vi "Memory.Error Handler.Replace String in Source.vi"(9 "offset (0)":i32, 10 "string":string, 11 "error in":errorcluster) -> (1 "new offset":i32, 3 "error out":errorcluster)   [LabVIEW 2016, in "LabVIEW Memory Manager.lvlib"]
uses:
  LabVIEW Memory Manager.lvlib
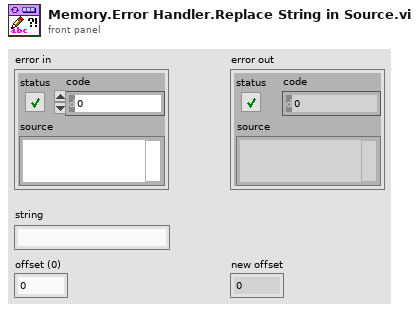
[diagram p1: front panel]
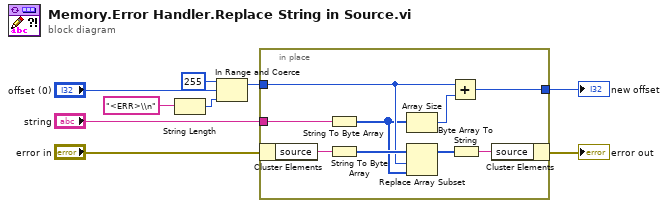
[diagram p0: block diagram]
diagram:
  n1 = String Length(string="<ERR>\\n") -> (length=w4:i32)
  n2 = In Range and Coerce(upper limit=255, x="offset (0)", lower limit=w4) -> (coerced(x)=w1:i32)  [unwired: 1 out]
  n3 = in-place {
    in-place-border: "string" -> [w15]
    in-place-border: w1 -> [w13]
    in-place-border: [w10] -> w6
    n4 = in-place-cluster #1("error in") -> ("source"=w17:string)
    n5 = String To Byte Array(string=w15) -> (unsigned byte array=w12:u8[])
    n6 = String To Byte Array(string=w17) -> (unsigned byte array=w16:u8[])
    n7 = Array Size(array=w12) -> (size(s)=w11:i32)
    n8 = Replace Array Subset(array=w16, new element=w12, index=w13) -> (w14:u8[])
    n9 = Add(x=w13, y=w11) -> (x+y=w10:i32)
    n10 = Byte Array To String(unsigned byte array=w14) -> (string=w18:string)
    n11 = in-place-cluster #1("source"=w18) -> (→"error out":errorcluster)
  }
  "new offset" <- w6
